vi "slider tabs open.vi"(10 "slider tab Ctrl Ref Name":string, 11 "close(T)/open(F)":bool) -> ()   [LabVIEW 2012]
doc: "This VI moves all slider tabs to the open position.\n\nIt can also be used to read the open position, should it ever get lost from the settings.ini."
uses:
  GFG/GFGfpRefGet.vi
  GFG/GFGnumericGet.vi
  GFG/GFG library.lvlib
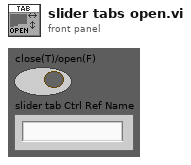
[diagram p1: front panel]
types:
  T1 = cluster{"WaveformChartRef":refnum<vi>, "DigitalRef":refnum<vi>, "ArrayRef":refnum<vi>, "TabControlRef":refnum<vi>, "EnumRef":refnum<vi>, "RingRef":refnum<vi>, "BooleanRef":refnum<vi>, "KnobRef":refnum<vi>, "SlideRef":refnum<vi>, "PathRef":refnum<vi>, "StringRef":refnum<vi>, "ComboBox":refnum<vi>, "WaveformGraphRef":refnum<vi>}
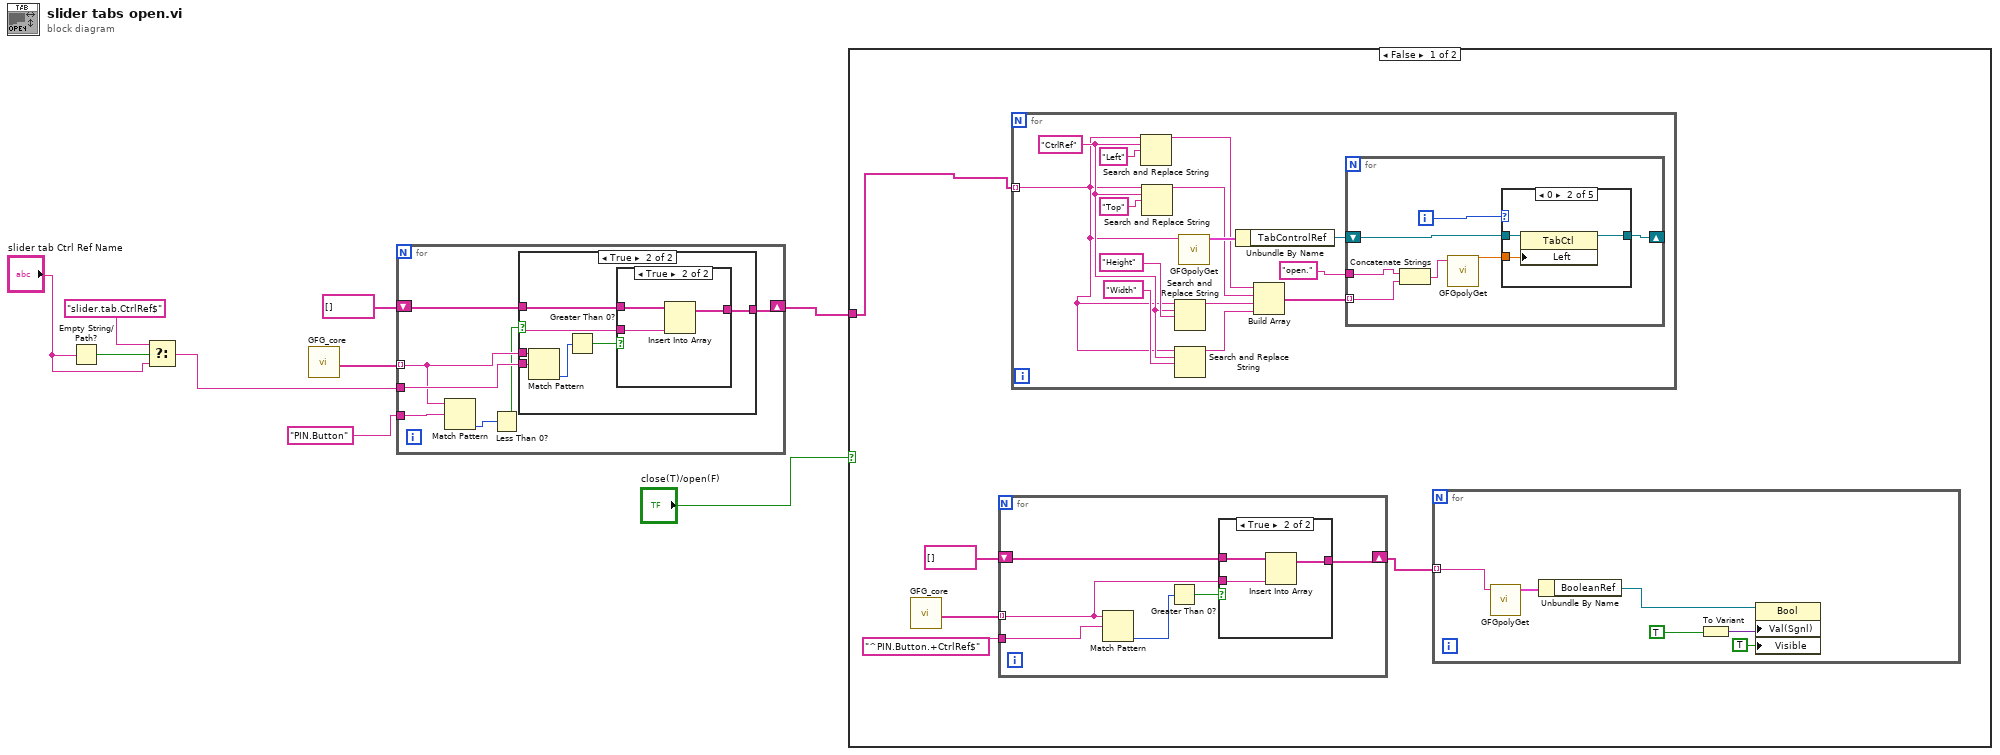
[diagram p0: block diagram]
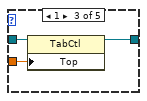
[diagram p3: hidden frame]
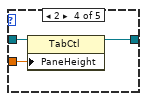
[diagram p4: hidden frame]
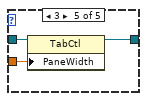
[diagram p5: hidden frame]
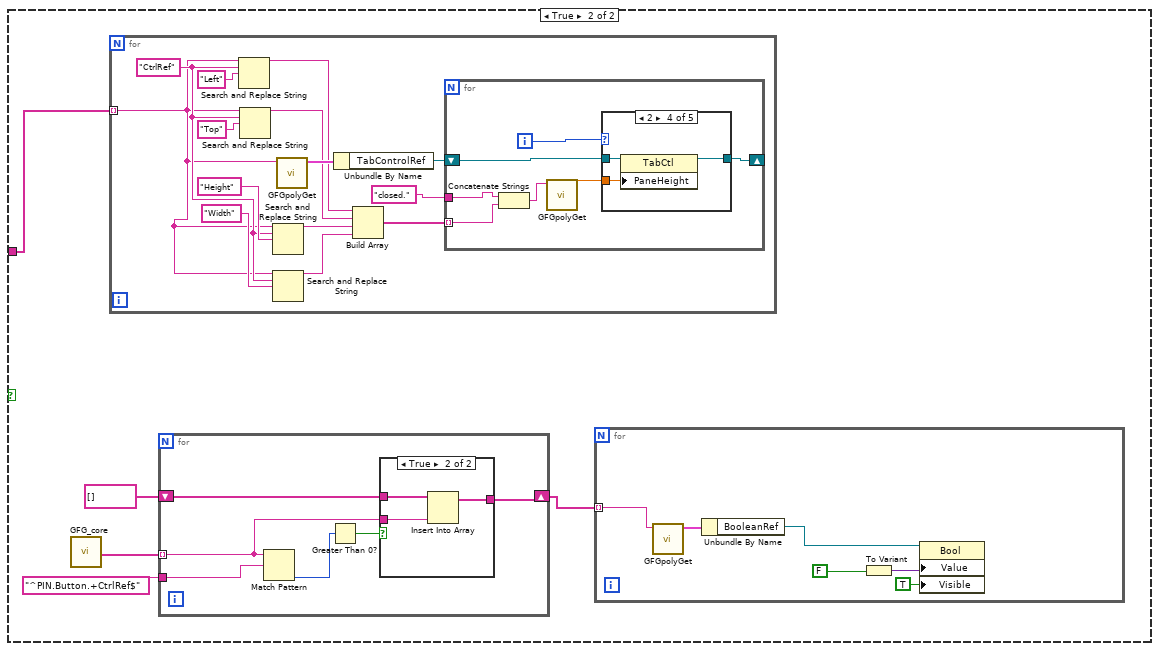
[diagram p7: hidden frame]
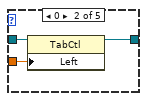
[diagram p9: hidden frame]
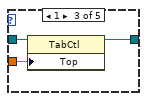
[diagram p10: hidden frame]
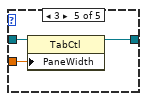
[diagram p11: hidden frame]
diagram:
  n1 = Empty String/Path?(string/path="slider tab Ctrl Ref Name") -> (empty?=w4:bool)
  n2 = Select(t="slider.tab.CtrlRef$" ("regular expression"), s=w4, f="slider tab Ctrl Ref Name") -> (s? t:f=w2:string)
  n3 = call "GFG_core.vi"() -> ("All Variable Names Out"=w9:string[])  [unwired: 13 in, 6 out]
  n4 = for {
    tunnel: w9 -> [w12] mode=indexing
    shift-right: [w15] -> w7
    shift-left: string[] [] ("All Variable Names Out") -> [w16]
    tunnel: w2 -> [w14]
    tunnel: "PIN.Button" ("regular expression") -> [w13]
    n5 = Match Pattern(string=w12, regular expression=w13) -> (offset past match=w11:i32)  [unwired: 1 in, 3 out]
    n6 = Less Than 0?(x=w11) -> (x < 0?=w10:bool)
    n7 = case shown="True" w10 {
      tunnel: w16 -> [w17 w22]
      tunnel: [w17 w21] -> w15
      tunnel: w14 -> [_ w19]
      tunnel: w12 -> [_ w18]
      frame False {
      }
      frame True {
        n8 = Match Pattern(string=w18, regular expression=w19) -> (offset past match=w23:i32)  [unwired: 1 in, 3 out]
        n9 = Greater Than 0?(x=w23) -> (x > 0?=w20:bool)
        n10 = case shown="True" w20 {
          tunnel: w22 -> [w24 w27]
          tunnel: [w24 w26] -> w21
          tunnel: w18 -> [_ w25]
          frame False {
          }
          frame True {
            n11 = Insert Into Array(array=w27, new element=w25) -> (w26:string[])  [unwired: 1 in]
          }
        }
      }
    }
  }
  n12 = case shown="False" "close(T)/open(F)" {
    tunnel: w7 -> [w28 w83]
    frame False {
      n13 = call "GFG_core.vi"() -> ("All Variable Names Out"=w30:string[])  [unwired: 13 in, 6 out]
      n14 = for {
        tunnel: w30 -> [w73] mode=indexing
        shift-right: [w76] -> w29
        shift-left: string[] [] ("All Variable Names Out") -> [w77]
        tunnel: "^PIN.Button.+CtrlRef$" ("regular expression") -> [w74]
        n15 = Match Pattern(string=w73, regular expression=w74) -> (offset past match=w78:i32)  [unwired: 1 in, 3 out]
        n16 = Greater Than 0?(x=w78) -> (x > 0?=w75:bool)
        n17 = case shown="True" w75 {
          tunnel: w77 -> [w79 w82]
          tunnel: [w79 w81] -> w76
          tunnel: w73 -> [_ w80]
          frame False {
          }
          frame True {
            n18 = Insert Into Array(array=w82, new element=w80) -> (w81:string[])  [unwired: 1 in]
          }
        }
      }
      n19 = for {
        tunnel: w28 -> [w35] mode=indexing
        w36 = "CtrlRef" ("search string")
        n20 = Search and Replace String(input string=w35, search string=w36, replace string="Left" ("replace string (\"\")")) -> (result string=w41:string)  [unwired: 5 in, 3 out]
        n21 = Search and Replace String(input string=w35, search string=w36, replace string="Top" ("replace string (\"\")")) -> (result string=w40:string)  [unwired: 5 in, 3 out]
        n22 = Search and Replace String(input string=w35, search string=w36, replace string="Height" ("replace string (\"\")")) -> (result string=w39:string)  [unwired: 5 in, 3 out]
        n23 = Search and Replace String(input string=w35, search string=w36, replace string="Width" ("replace string (\"\")")) -> (result string=w38:string)  [unwired: 5 in, 3 out]
        n24 = call-poly "GFGpolyGet.vi"("Variable Name in"=w35) -> ("output cluster"=w46:T1)  [unwired: 9 in, 1 out]
        n25 = Unbundle By Name(w46) -> ("TabControlRef"=w34:refnum<vi>)
        n26 = Build Array(w41, w40, w39, w38) -> (w37:string[])
        n27 = for {
          tunnel: w37 -> [w48] mode=indexing
          shift-right: [w50] -> _
          shift-left: w34 -> [w51]
          tunnel: "open." ("element") -> [w49]
          i -> [w53]
          n28 = Concatenate Strings(w49, w48) -> (w47:string)
          n29 = call-poly "GFGpolyGet.vi"("Variable Name in"=w47) -> ("Numeric"=w52:dbl)  [unwired: 9 in, 1 out]
          n30 = case shown="0" w53 {
            tunnel: w52 -> [_ w57 w60 w63 w66]
            tunnel: w51 -> [w54 w56 w59 w62 w65]
            tunnel: [w54 w55 w58 w61 w64] -> w50
            frame -1, Default {
            }
            frame 0 {
              n31 = property class="TabCtl"(reference=w56, "Left"=w57) -> (reference out=w55:refnum<vi>)  [unwired: 1 in, 1 out]
            }
            frame 1 {
              n32 = property class="TabCtl"(reference=w59, "Top"=w60) -> (reference out=w58:refnum<vi>)  [unwired: 1 in, 1 out]
            }
            frame 2 {
              n33 = property class="TabCtl"(reference=w62, "PaneHeight"=w63) -> (reference out=w61:refnum<vi>)  [unwired: 1 in, 1 out]
            }
            frame 3 {
              n34 = property class="TabCtl"(reference=w65, "PaneWidth"=w66) -> (reference out=w64:refnum<vi>)  [unwired: 1 in, 1 out]
            }
          }
        }
      }
      n35 = for {
        tunnel: w29 -> [w70] mode=indexing
        n36 = call-poly "GFGpolyGet.vi"("Variable Name in"=w70) -> ("output cluster"=w72:T1)  [unwired: 9 in, 1 out]
        n37 = Unbundle By Name(w72) -> ("BooleanRef"=w71:refnum<vi>)
        n38 = To Variant(anything=TRUE ("Set(T)/Reset(F)")) -> (Variant=w69:variant)
        n39 = property class="Bool"(reference=w71, "Val(Sgnl)"=w69, "Visible"=TRUE) -> ()  [unwired: 1 in, 2 out]
      }
    }
    frame True {
      n40 = call "GFG_core.vi"() -> ("All Variable Names Out"=w85:string[])  [unwired: 13 in, 6 out]
      n41 = for {
        tunnel: w83 -> [w90] mode=indexing
        w91 = "CtrlRef" ("search string")
        n42 = Search and Replace String(input string=w90, search string=w91, replace string="Left" ("replace string (\"\")")) -> (result string=w96:string)  [unwired: 5 in, 3 out]
        n43 = Search and Replace String(input string=w90, search string=w91, replace string="Top" ("replace string (\"\")")) -> (result string=w95:string)  [unwired: 5 in, 3 out]
        n44 = Search and Replace String(input string=w90, search string=w91, replace string="Height" ("replace string (\"\")")) -> (result string=w94:string)  [unwired: 5 in, 3 out]
        n45 = Search and Replace String(input string=w90, search string=w91, replace string="Width" ("replace string (\"\")")) -> (result string=w93:string)  [unwired: 5 in, 3 out]
        n46 = call-poly "GFGpolyGet.vi"("Variable Name in"=w90) -> ("output cluster"=w101:T1)  [unwired: 9 in, 1 out]
        n47 = Unbundle By Name(w101) -> ("TabControlRef"=w89:refnum<vi>)
        n48 = Build Array(w96, w95, w94, w93) -> (w92:string[])
        n49 = for {
          tunnel: w92 -> [w103] mode=indexing
          shift-right: [w105] -> _
          shift-left: w89 -> [w106]
          tunnel: "closed." ("element") -> [w104]
          i -> [w108]
          n50 = Concatenate Strings(w104, w103) -> (w102:string)
          n51 = call-poly "GFGpolyGet.vi"("Variable Name in"=w102) -> ("Numeric"=w107:dbl)  [unwired: 9 in, 1 out]
          n52 = case shown="2" w108 {
            tunnel: w107 -> [_ w112 w115 w118 w121]
            tunnel: w106 -> [w109 w111 w114 w117 w120]
            tunnel: [w109 w110 w113 w116 w119] -> w105
            frame -1, Default {
            }
            frame 0 {
              n53 = property class="TabCtl"(reference=w111, "Left"=w112) -> (reference out=w110:refnum<vi>)  [unwired: 1 in, 1 out]
            }
            frame 1 {
              n54 = property class="TabCtl"(reference=w114, "Top"=w115) -> (reference out=w113:refnum<vi>)  [unwired: 1 in, 1 out]
            }
            frame 2 {
              n55 = property class="TabCtl"(reference=w117, "PaneHeight"=w118) -> (reference out=w116:refnum<vi>)  [unwired: 1 in, 1 out]
            }
            frame 3 {
              n56 = property class="TabCtl"(reference=w120, "PaneWidth"=w121) -> (reference out=w119:refnum<vi>)  [unwired: 1 in, 1 out]
            }
          }
        }
      }
      n57 = for {
        tunnel: w85 -> [w128] mode=indexing
        shift-right: [w131] -> w84
        shift-left: string[] [] ("All Variable Names Out") -> [w132]
        tunnel: "^PIN.Button.+CtrlRef$" ("regular expression") -> [w129]
        n58 = Match Pattern(string=w128, regular expression=w129) -> (offset past match=w133:i32)  [unwired: 1 in, 3 out]
        n59 = Greater Than 0?(x=w133) -> (x > 0?=w130:bool)
        n60 = case shown="True" w130 {
          tunnel: w132 -> [w134 w137]
          tunnel: [w134 w136] -> w131
          tunnel: w128 -> [_ w135]
          frame False {
          }
          frame True {
            n61 = Insert Into Array(array=w137, new element=w135) -> (w136:string[])  [unwired: 1 in]
          }
        }
      }
      n62 = for {
        tunnel: w84 -> [w125] mode=indexing
        n63 = call-poly "GFGpolyGet.vi"("Variable Name in"=w125) -> ("output cluster"=w127:T1)  [unwired: 9 in, 1 out]
        n64 = Unbundle By Name(w127) -> ("BooleanRef"=w126:refnum<vi>)
        n65 = To Variant(anything=FALSE ("Set(T)/Reset(F)")) -> (Variant=w124:variant)
        n66 = property class="Bool"(reference=w126, "Value"=w124, "Visible"=TRUE) -> ()  [unwired: 1 in, 2 out]
      }
    }
  }
